vi "Example_sequence_acquisition.vi"() -> ()   [LabVIEW 2021]
uses:
  src/Low_level_subVIs/PVCAM_rgn_type.ctl
panel:
  out "Image":dbl[][](graph)
  out "return type":i16
  out "bytes_remaining":u32
  out "return uninit":i16
  in  "exp_time":u16=100
  out "return type 3":i16
  out "Sensor temperature":i16
  out "error code":i16
  out "return out 2":i16
  out "return value 2":i16
  out "string":string
  out "return out":i16
  out "hCam out":i16
  out "return value":i16
  out "error out":errorcluster
  in  "error in (no error)":errorcluster
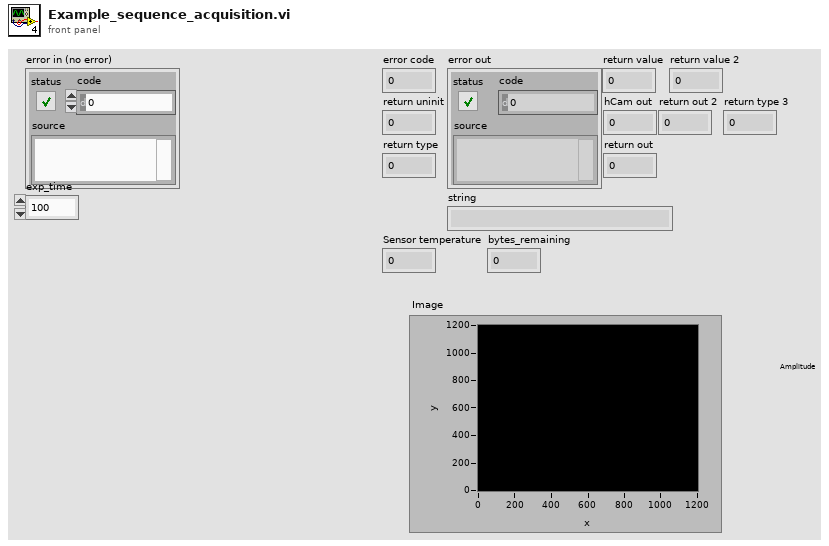
[diagram p1: front panel]
types:
  T1 = typedef "PVCAM_rgn_type.ctl" = cluster{"s1":u16, "s2":u16, "sbin":u16, "p1":u16, "p2":u16, "pbin":u16}
  T2 = enum16{"ATTR_CURRENT", "ATTR_COUNT", "ATTR_TYPE", "ATTR_MIN", "ATTR_MAX", "ATTR_DEFAULT", "ATTR_INCREMENT", "ATTR_ACCESS", "ATTR_AVAIL"}
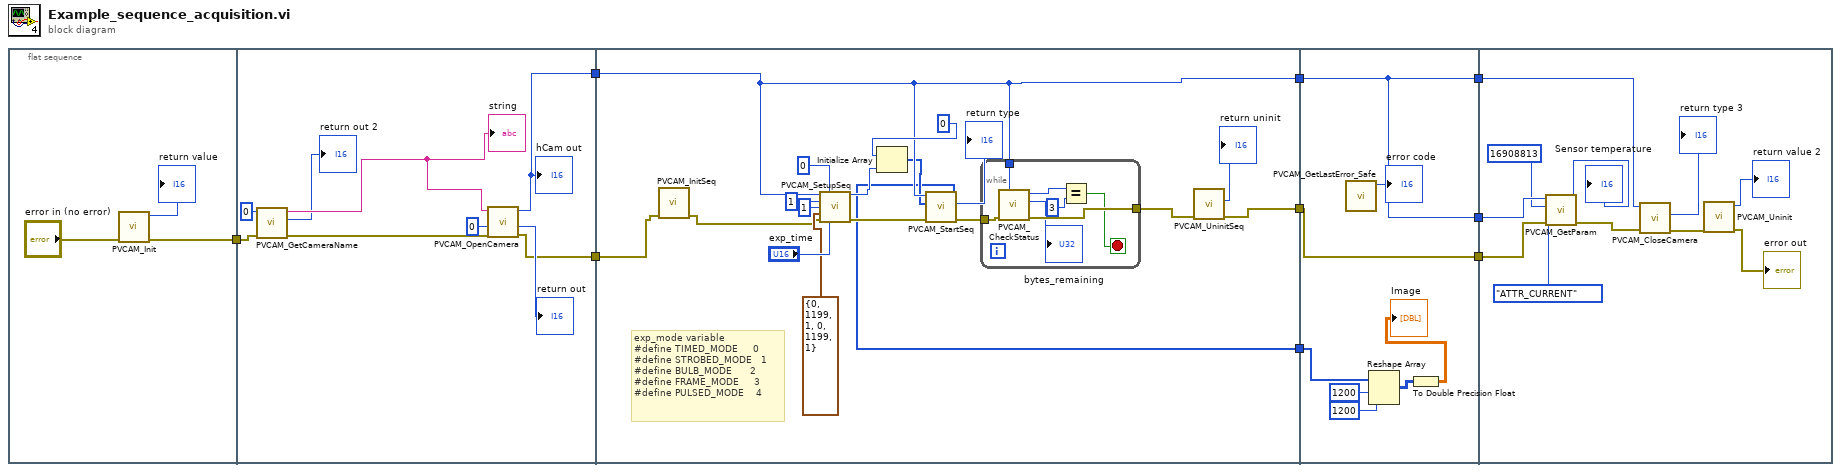
[diagram p0: block diagram]
diagram:
  n1 = flat-sequence {
    tunnel: [w11] -> w9
    tunnel: w9 -> [w15]
    tunnel: [w14] -> w6
    tunnel: [w13] -> w5
    tunnel: w6 -> [w33]
    tunnel: w5 -> [w28]
    tunnel: [w28] -> w4
    tunnel: [w25] -> w2
    tunnel: [w22] -> w1
    tunnel: [w52] -> w8
    tunnel: [w53] -> w7
    tunnel: w4 -> [w53]
    tunnel: [w53] -> w3
    tunnel: w2 -> [w52]
    tunnel: w1 -> [w51]
    tunnel: w8 -> [w63]
    tunnel: w7 -> [w62]
    tunnel: w3 -> [w58]
    frame #0 {
      n2 = call "PVCAM_Init.vi"("error in (no error)"="error in (no error)") -> ("error out"=w11:errorcluster, "return value"=→"return value":i16)  [unwired: 9 in]
    }
    frame #1 {
      n3 = call "PVCAM_GetCameraName.vi"("error in (no error)"=w15, "index in"=i16 0) -> ("error out"=w20:errorcluster, "return out"=→"return out 2":i16, "string"=w21:string)  [unwired: 6 in, 1 out]
      "string" <- w21
      n4 = call "PVCAM_OpenCamera.vi"("error in (no error)"=w20, "mode"=i16 0, "cameraName"=w21) -> ("error out"=w14:errorcluster, "return out"=→"return out":i16, "hCam out"=w13:i16)  [unwired: 6 in]
      "hCam out" <- w13
    }
    frame #2 {
      # "exp_mode variable\n#define TIMED_MODE     0\n#define STROBED_MODE   1\n#define BULB_MODE      2\n#define FRAME_MODE     3\n#define PULSED_MODE    4"
      n5 = call "PVCAM_InitSeq.vi"("error in (no error)"=w33) -> ("error out"=w34:errorcluster)  [unwired: 9 in, 1 out]
      n6 = call "PVCAM_SetupSeq.vi"("hCam"=w28, "exp_mode"=i16 0, "exp_total"=u16 1, "rgn_total"=i16 1, "rgn_type"=T1 {"s1"=0, "s2"=1199, "sbin"=1, "p1"=0, "p2"=1199, "pbin"=1}, "error in (no error)"=w34, "exp_time"="exp_time") -> ("stream_size"=w31:u32, "error out"=w32:errorcluster)  [unwired: 6 in, 1 out]
      n7 = Initialize Array(u8 0 ("element"), w31) -> (w27:u8[])
      n8 = call "PVCAM_StartSeq.vi"("error in (no error)"=w32, "buffer"=w27, "hCam"=w28) -> ("error out"=w29:errorcluster, "return type"=→"return type":i16, "ImageBuf"=w22:u16[])  [unwired: 6 in]
      n9 = while {
        tunnel: w29 -> [w46]
        tunnel: [w45] -> w26
        tunnel: w28 -> [w44]
        stop <- w41 stop-if-true
        n10 = call "PVCAM_CheckStatus.vi"("error in (no error)"=w46, "hCam"=w44) -> ("error out"=w45:errorcluster, "bytes_remaining"=→"bytes_remaining":u32, "status"=w43:i16)  [unwired: 7 in]
        n11 = Equal?(x=w43, y=i16 3) -> (x = y?=w41:bool)
      }
      n12 = call "PVCAM_UninitSeq.vi"("error in (no error)"=w26) -> ("error out"=w25:errorcluster, "return"=→"return uninit":i16)  [unwired: 9 in]
    }
    frame #3 {
      n13 = call "PVCAM_GetLastError_Safe.vi"() -> ("return type"=→"error code":i16)  [unwired: 11 in]
      n14 = Reshape Array(w51, 1200 ("dimension size"), 1200 ("dimension size")) -> (w48:u16[][])
      n15 = To Double Precision Float(number=w48) -> (double precision float=→"Image":dbl[][])
    }
    frame #4 {
      n16 = call "PVCAM_GetParam.vi"("error in (no error)"=w63, "param_attrib"=T2."ATTR_CURRENT", "param_id"=u32 16908813, "hCam"=w62) -> ("error out"=w61:errorcluster, "param_value"=→"Sensor temperature":i16)  [unwired: 5 in, 1 out]
      n17 = call "PVCAM_CloseCamera.vi"("error in (no error)"=w61, "hCam"=w58) -> ("error out"=w60:errorcluster, "return type 2"=→"return type 3":i16)  [unwired: 8 in]
      n18 = call "PVCAM_Uninit.vi"("error in (no error)"=w60) -> ("error out"=→"error out":errorcluster, "return value"=→"return value 2":i16)  [unwired: 9 in]
    }
  }
